vi "Utility Write Config INI to File.vi"(6 "File Name":string, 7 "File Type":string(combo)=".ini", 8 "Error In":errorcluster, 10 "reference":refnum<vi>, 11 "Path In":path) -> (0 "Error Out":errorcluster, 3 "Path Out":path)   [LabVIEW 2015]
uses:
  <vilib>/Utility/config.llb/Write Key (String).vi
  <vilib>/Utility/config.llb/NI_LVConfig.lvlib
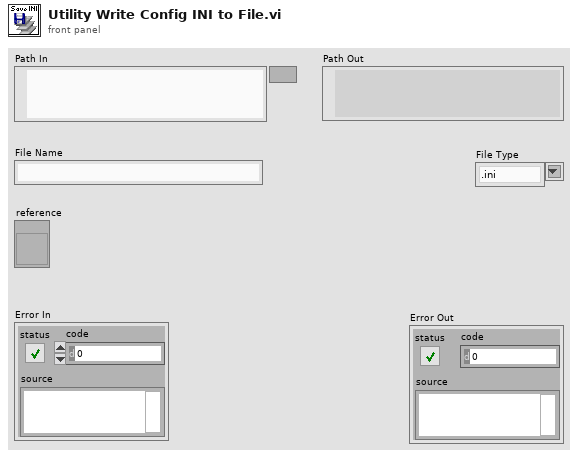
[diagram p1: front panel]
types:
  T1 = typedef "NI_LVConfig.lvlib/Config Data RefNum.ctl" = refnum<k1>
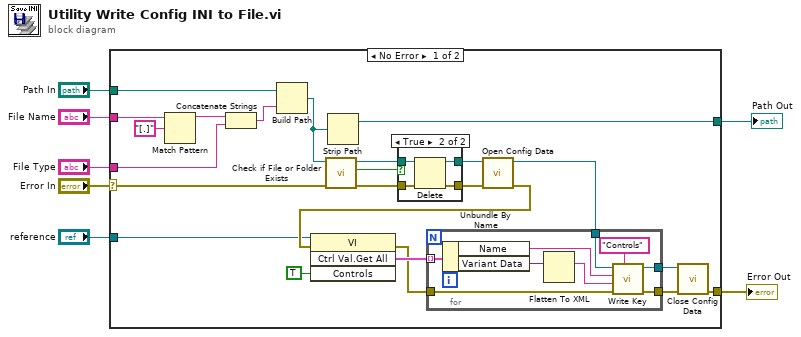
[diagram p0: block diagram]
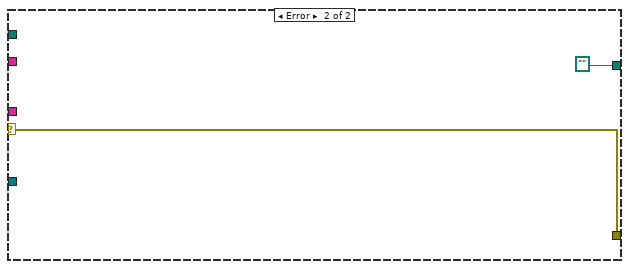
[diagram p3: hidden frame]
diagram:
  n1 = case shown="No Error" "Error In" {
    selector: "Error In" -> [w22 w47]
    tunnel: [w15 w47] -> w2
    tunnel: [w8 path ""] -> w7
    tunnel: "Path In" -> [w11 _]
    tunnel: "File Type" -> [w13 _]
    tunnel: "reference" -> [w12 _]
    tunnel: "File Name" -> [w10 _]
    frame No Error {
      n2 = Match Pattern(string=w10, regular expression="[.]" ("search string")) -> (before substring=w28:string)  [unwired: 1 in, 3 out]
      n3 = Concatenate Strings(w28, w13) -> (w27:string)
      n4 = Build Path(base path=w11, name or relative path=w27) -> (appended path=w9:path)
      n5 = call <vilib>:"Check if File or Folder Exists.vi"("error in (no error)"=w22, "path"=w9) -> ("error out"=w25:errorcluster, "file or folder exists?"=w26:bool, "dup path"=w14:path)  [unwired: 7 in]
      n6 = Strip Path(path=w9) -> (stripped path=w8:path)  [unwired: 1 out]
      n7 = case shown="True" w26 {
        tunnel: w25 -> [w40 w45]
        tunnel: w14 -> [w41 w44]
        tunnel: [w41 w43] -> w24
        tunnel: [w40 w42] -> w23
        frame False {
        }
        frame True {
          n8 = Delete(path (use dialog)=w44, error in=w45) -> (deleted path=w43:path, error out=w42:errorcluster)  [unwired: 3 in, 1 out]
        }
      }
      n9 = call <vilib>:"Open Config Data.vi"("error in (no error)"=w23, "configuration file path"=w24) -> ("error out"=w19:errorcluster, "refnum"=w20:T1)  [unwired: 1 in, 7 out]
      n10 = invoke class="VI" method="Ctrl Val.Get All"(reference=w12, error in=w19, "Controls"=TRUE) -> (error out=w18:errorcluster, "Get All Control Values Variant"=w21:cluster{"Name":string, "Variant Data":variant}[])  [unwired: 1 in, 2 out]
      n11 = for {
        tunnel: w21 -> [w39] mode=indexing
        tunnel: w20 -> [w36]
        tunnel: w18 -> [w35]
        tunnel: [w32] -> w17
        tunnel: [w31] -> w16
        n12 = Unbundle By Name(w39) -> ("Name"=w34:string, "Variant Data"=w38:variant)
        n13 = Flatten To XML(anything=w38) -> (xml string=w33:string)
        n14 = call-poly <vilib>:"Write Key.vi"("section"="Controls", "error in (no error)"=w35, "value"=w33, "key"=w34, "refnum"=w36) -> ("error out"=w31:errorcluster, "refnum out"=w32:T1)  [unwired: 4 in, 1 out]
      }
      n15 = call <vilib>:"Close Config Data.vi"("error in (no error)"=w16, "refnum"=w17) -> ("error out"=w15:errorcluster)  [unwired: 1 in, 8 out]
    }
    frame Error {
      (unwired) ""
    }
  }
  "Path Out" <- w7
  "Error Out" <- w2
